vi "parse-status(x).vi"(1 "Writein the response of the ps180 to the Status command (X):":string) -> (0 "Status":string)   [LabVIEW 2024]
panel:
  in  "Pn":string[](array[string])=["Output Clamped (Transition))", "Forward (Verification)", "Reverse (Verification)", "", "Output Clamped (Requested)"]
  in  "Pm":string[](array[string])=["set point=Forward, last persistent=Forward, present=Forward", "set point=Forward, last persistent=Forward, present=Reverse", "set point=Forward, last persistent=Reverse, present=Forward", "set point=Forward, last persistent=Reverse, present=Reverse", "set point=Reverse, last persistent=Forward, present=Forward", "set point=Reverse, last persistent=Forward, present=Reverse", "set point=Reverse, last persistent=Reverse, present=Forward", "set point=Reverse, last persistent=Reverse, present=Reverse"]
  in  "Mn":string[](array[string])=["at Rest (output constant)", "Sweeping (output changing)", "Rate limiting (output changing)", "Sweeping & Rate limiting (output changing)"]
  in  "Mm":string[](array[string])=["display=Amps, mode=Immediate, magnet sweep=Fast", "display=Tesla, mode=Immediate, magnet sweep=Fast", "display=Amps, mode=Sweep, magnet sweep=Fast", "display=Tesla, mode=Sweep, magnet sweep=Fast", "display=Amps, mode=Immediate, magnet sweep=Train", "display=Tesla, mode=Immediate, magnet sweep=Train", "display=Amps, mode=Sweep, magnet sweep=Train", "display=Tesla, mode=Sweep, magnet sweep=Train"]
  in  "Hn":string[](array[string])=["Off (Magnet @ zero)", "On", "Off (magnet @ field)", "", "", "", "", "", "No switch fitted"]
  in  "Cn":string[](array[string])=["Local (locked)", "Remote (locked)", "Local", "Remote", "Auto-Run-Down", "Auto-Run-Down", "Auto-Run-Down", "Auto-Run-Down"]
  in  "An":string[](array[string])=["at Hold", "to Set point", "to Zero", "", "Clamped"]
  in  "Xn description":string[](array[string])=["Normal", "On +ve voltage limit", "On -ve voltage limit", "", "Outside -ve current limit", "", "", "", "Outside +ve current limit"]
  in  "Xm description":string[](array[string])=["Normal", "Quenched", "Over heated", "", "Warming up"]
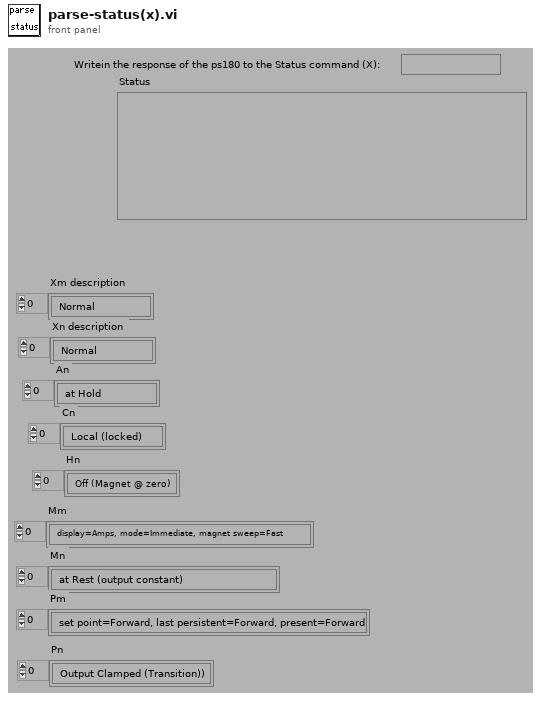
[diagram p1: front panel]
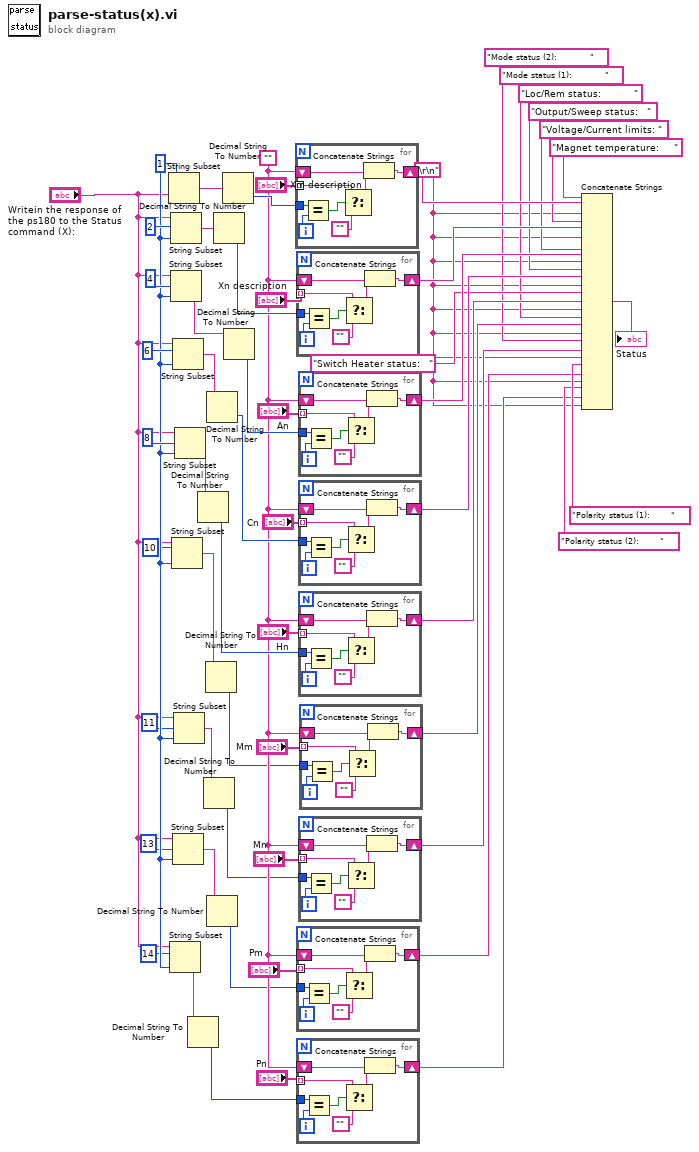
[diagram p0: block diagram]
diagram:
  w2 = "\r\n"
  w28 = ""
  w23 = 1
  n1 = String Subset(string="Writein the response of the ps180 to the Status command (X):", offset (0)=w23, length (rest)=w23) -> (substring=w58:string)
  n2 = String Subset(string="Writein the response of the ps180 to the Status command (X):", offset (0)=14, length (rest)=w23) -> (substring=w13:string)
  n3 = String Subset(string="Writein the response of the ps180 to the Status command (X):", offset (0)=2, length (rest)=w23) -> (substring=w53:string)
  n4 = String Subset(string="Writein the response of the ps180 to the Status command (X):", offset (0)=4, length (rest)=w23) -> (substring=w44:string)
  n5 = String Subset(string="Writein the response of the ps180 to the Status command (X):", offset (0)=10, length (rest)=w23) -> (substring=w18:string)
  n6 = String Subset(string="Writein the response of the ps180 to the Status command (X):", offset (0)=6, length (rest)=w23) -> (substring=w36:string)
  n7 = String Subset(string="Writein the response of the ps180 to the Status command (X):", offset (0)=13, length (rest)=w23) -> (substring=w14:string)
  n8 = String Subset(string="Writein the response of the ps180 to the Status command (X):", offset (0)=11, length (rest)=w23) -> (substring=w17:string)
  n9 = String Subset(string="Writein the response of the ps180 to the Status command (X):", offset (0)=8, length (rest)=w23) -> (substring=w35:string)
  n10 = Decimal String To Number(string=w13) -> (number=w11:i32)  [unwired: 2 in, 1 out]
  n11 = Decimal String To Number(string=w35) -> (number=w33:i32)  [unwired: 2 in, 1 out]
  n12 = Decimal String To Number(string=w17) -> (number=w15:i32)  [unwired: 2 in, 1 out]
  n13 = Decimal String To Number(string=w18) -> (number=w16:i32)  [unwired: 2 in, 1 out]
  n14 = Decimal String To Number(string=w36) -> (number=w34:i32)  [unwired: 2 in, 1 out]
  n15 = Decimal String To Number(string=w14) -> (number=w12:i32)  [unwired: 2 in, 1 out]
  n16 = Decimal String To Number(string=w53) -> (number=w52:i32)  [unwired: 2 in, 1 out]
  n17 = Decimal String To Number(string=w58) -> (number=w57:i32)  [unwired: 2 in, 1 out]
  n18 = Decimal String To Number(string=w44) -> (number=w43:i32)  [unwired: 2 in, 1 out]
  n19 = for {
    tunnel: w57 -> [w66]
    shift-right: [w62] -> w51
    shift-left: w28 -> [w63]
    tunnel: "Xm description" -> [w61] mode=indexing
    i -> [w65]
    n20 = Equal?(x=w66, y=w65) -> (x = y?=w64:bool)
    n21 = Select(t=w61, s=w64, f="") -> (s? t:f=w59:string)
    n22 = Concatenate Strings(w63, w59) -> (w62:string)
  }
  n23 = for {
    tunnel: w52 -> [w74]
    shift-right: [w70] -> w48
    shift-left: w28 -> [w71]
    tunnel: "Xn description" -> [w69] mode=indexing
    i -> [w73]
    n24 = Equal?(x=w74, y=w73) -> (x = y?=w72:bool)
    n25 = Select(t=w69, s=w72, f="") -> (s? t:f=w67:string)
    n26 = Concatenate Strings(w71, w67) -> (w70:string)
  }
  n27 = for {
    shift-right: [w79] -> w5
    shift-left: w28 -> [w80]
    tunnel: "Pm" -> [w78] mode=indexing
    tunnel: w12 -> [w75]
    i -> [w82]
    n28 = Equal?(x=w75, y=w82) -> (x = y?=w81:bool)
    n29 = Select(t=w78, s=w81, f="") -> (s? t:f=w76:string)
    n30 = Concatenate Strings(w80, w76) -> (w79:string)
  }
  n31 = for {
    shift-right: [w87] -> w3
    shift-left: w28 -> [w88]
    tunnel: "Pn" -> [w86] mode=indexing
    tunnel: w11 -> [w83]
    i -> [w90]
    n32 = Equal?(x=w83, y=w90) -> (x = y?=w89:bool)
    n33 = Select(t=w86, s=w89, f="") -> (s? t:f=w84:string)
    n34 = Concatenate Strings(w88, w84) -> (w87:string)
  }
  n35 = for {
    shift-right: [w95] -> w41
    shift-left: w28 -> [w96]
    tunnel: "An" -> [w94] mode=indexing
    tunnel: w43 -> [w91]
    i -> [w98]
    n36 = Equal?(x=w91, y=w98) -> (x = y?=w97:bool)
    n37 = Select(t=w94, s=w97, f="") -> (s? t:f=w92:string)
    n38 = Concatenate Strings(w96, w92) -> (w95:string)
  }
  n39 = for {
    shift-right: [w103] -> w31
    shift-left: w28 -> [w104]
    tunnel: "Cn" -> [w102] mode=indexing
    tunnel: w34 -> [w99]
    i -> [w106]
    n40 = Equal?(x=w99, y=w106) -> (x = y?=w105:bool)
    n41 = Select(t=w102, s=w105, f="") -> (s? t:f=w100:string)
    n42 = Concatenate Strings(w104, w100) -> (w103:string)
  }
  n43 = for {
    shift-right: [w111] -> w29
    shift-left: w28 -> [w112]
    tunnel: "Hn" -> [w110] mode=indexing
    tunnel: w33 -> [w107]
    i -> [w114]
    n44 = Equal?(x=w107, y=w114) -> (x = y?=w113:bool)
    n45 = Select(t=w110, s=w113, f="") -> (s? t:f=w108:string)
    n46 = Concatenate Strings(w112, w108) -> (w111:string)
  }
  n47 = for {
    shift-right: [w119] -> w7
    shift-left: w28 -> [w120]
    tunnel: "Mn" -> [w118] mode=indexing
    tunnel: w15 -> [w115]
    i -> [w122]
    n48 = Equal?(x=w115, y=w122) -> (x = y?=w121:bool)
    n49 = Select(t=w118, s=w121, f="") -> (s? t:f=w116:string)
    n50 = Concatenate Strings(w120, w116) -> (w119:string)
  }
  n51 = for {
    shift-right: [w127] -> w9
    shift-left: w28 -> [w128]
    tunnel: "Mm" -> [w126] mode=indexing
    tunnel: w16 -> [w123]
    i -> [w130]
    n52 = Equal?(x=w123, y=w130) -> (x = y?=w129:bool)
    n53 = Select(t=w126, s=w129, f="") -> (s? t:f=w124:string)
    n54 = Concatenate Strings(w128, w124) -> (w127:string)
  }
  n55 = Concatenate Strings("Magnet temperature:     ", w51, w2, "Voltage/Current limits: ", w48, w2, "Output/Sweep status:   ", w41, w2, "Loc/Rem status:           ", w31, w2, "Switch Heater status:   ", w29, w2, "Mode status (1):           ", w9, w2, "Mode status (2):           ", w7, w2, "Polarity status (1):       ", w5, w2, "Polarity status (2):       ", w3, w2) -> (→"Status":string)
